vi "dropdown.vi"(9 "side":enum16{"l", "r"}(ring)) -> ()   [LabVIEW 2017]
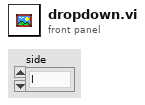
[diagram p1: front panel]
types:
  T1 = enum16{"hold", "f", "fl", "fr", "l", "r", "b", "bl", "br"}
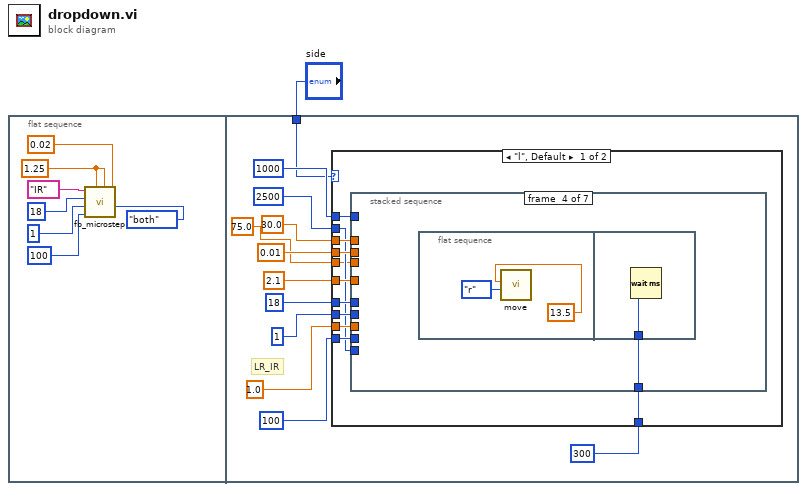
[diagram p0: block diagram]
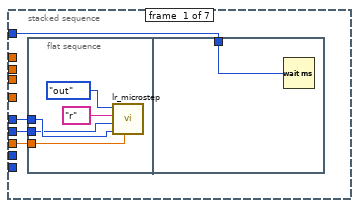
[diagram p2: hidden frame]
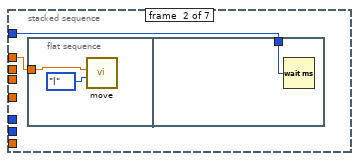
[diagram p3: hidden frame]
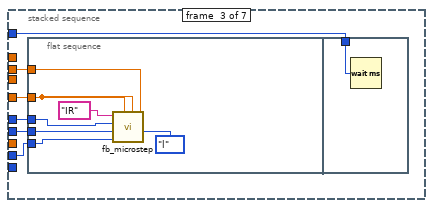
[diagram p4: hidden frame]
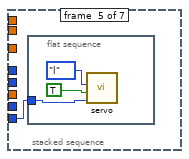
[diagram p5: hidden frame]
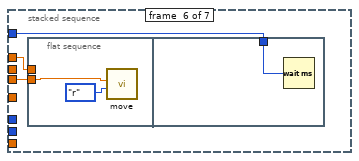
[diagram p6: hidden frame]
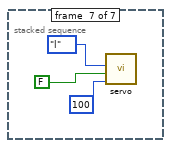
[diagram p7: hidden frame]
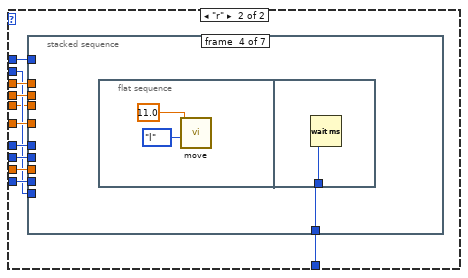
[diagram p8: hidden frame]
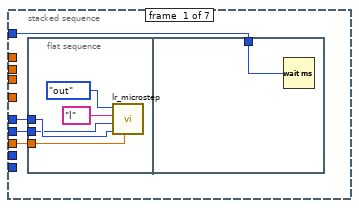
[diagram p9: hidden frame]
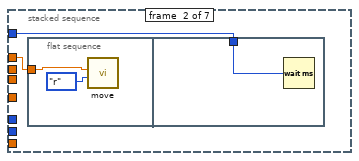
[diagram p10: hidden frame]
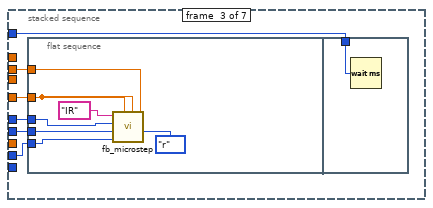
[diagram p11: hidden frame]
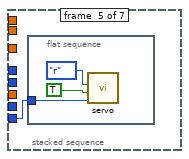
[diagram p12: hidden frame]
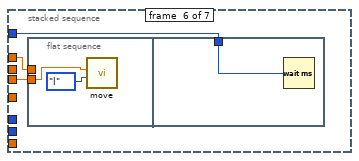
[diagram p13: hidden frame]
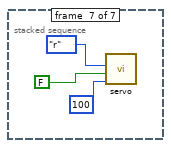
[diagram p14: hidden frame]
diagram:
  n1 = flat-sequence {
    tunnel: "side" -> [w11]
    frame #0 {
      w8 = 1.25 ("taget_IR_R")
      n2 = call "fb_microstep.vi"("Sensor"=enum16{"l", "r", "both"}."both", "precision"=0.02, "taget_IR_L"=w8, "taget_IR_R"=w8, "SamplingNUM"=100, "Step"=1, "Delay"=18, "Stop Mode"="IR") -> ()  [unwired: 3 in, 1 out]
    }
    frame #1 {
      # "LR_IR"
      n3 = case shown="\"l\", Default" w11 {
        tunnel: 18 ("Delay") -> [w31 w88]
        tunnel: 1 ("Step") -> [w30 w87]
        tunnel: 1.0 ("logic_num") -> [w29 w86]
        tunnel: 30.0 ("D") -> [w28 w85]
        tunnel: 2.1 ("taget_IR_R") -> [w27 w84]
        tunnel: 0.01 ("precision") -> [w26 w83]
        tunnel: 100 ("SamplingNUM") -> [w25 w82]
        tunnel: u32 1000 ("milliseconds to wait") -> [w24 w81]
        tunnel: u32 2500 ("delay") -> [w23 w80]
        tunnel: u32 300 ("milliseconds to wait") -> [w22 w79]
        tunnel: 75.0 ("D") -> [w21 w78]
        frame "l", Default {
          n4 = stacked-sequence {
            tunnel: w31 -> [w35 _ w50 _ _ _ _]
            tunnel: w30 -> [w34 _ w49 _ _ _ _]
            tunnel: w29 -> [w33 _ _ _ _ _ _]
            tunnel: w28 -> [_ w43 _ _ _ w71 _]
            tunnel: w27 -> [_ _ w52 _ _ _ _]
            tunnel: w26 -> [_ _ w51 _ _ _ _]
            tunnel: w25 -> [_ _ w48 _ _ _ _]
            tunnel: w24 -> [w32 w42 w47 _ _ w70 _]
            tunnel: w23 -> [_ _ _ _ w65 _ _]
            tunnel: w22 -> [_ _ _ w61 _ _ _]
            tunnel: w21 -> [_ _ _ _ _ w69 _]
            frame #0 {
              n5 = flat-sequence {
                tunnel: w35 -> [w38]
                tunnel: w34 -> [w37]
                tunnel: w33 -> [w36]
                tunnel: w32 -> [w41]
                frame #0 {
                  n6 = call "lr_microstep.vi"("target_IR"=w36, "Delay"=w38, "Step"=w37, "Stop Mode"="r", "IN-OUT"=enum16{"out", "in"}."out") -> ()  [unwired: 6 in, 1 out]
                }
                frame #1 {
                  n7 = Wait (ms)(milliseconds to wait=w41) -> ()  [unwired: 1 out]
                }
              }
            }
            frame #1 {
              n8 = flat-sequence {
                tunnel: w43 -> [w44]
                tunnel: w42 -> [w46]
                frame #0 {
                  n9 = call "move.vi"("Enum"=T1."l", "D"=w44) -> ()  [unwired: 10 in]
                }
                frame #1 {
                  n10 = Wait (ms)(milliseconds to wait=w46) -> ()  [unwired: 1 out]
                }
              }
            }
            frame #2 {
              n11 = flat-sequence {
                tunnel: w52 -> [w57]
                tunnel: w51 -> [w56]
                tunnel: w50 -> [w55]
                tunnel: w49 -> [w54]
                tunnel: w48 -> [w53]
                tunnel: w47 -> [w60]
                frame #0 {
                  n12 = call "fb_microstep.vi"("Sensor"=enum16{"l", "r", "both"}."l", "precision"=w56, "taget_IR_L"=w57, "taget_IR_R"=w57, "SamplingNUM"=w53, "Step"=w54, "Delay"=w55, "Stop Mode"="IR") -> ()  [unwired: 3 in, 1 out]
                }
                frame #1 {
                  n13 = Wait (ms)(milliseconds to wait=w60) -> ()  [unwired: 1 out]
                }
              }
            }
            frame #3 {
              n14 = flat-sequence {
                tunnel: w61 -> [w64]
                frame #0 {
                  n15 = call "move.vi"("Enum"=T1."r", "D"=13.5) -> ()  [unwired: 10 in]
                }
                frame #1 {
                  n16 = Wait (ms)(milliseconds to wait=w64) -> ()  [unwired: 1 out]
                }
              }
            }
            frame #4 {
              n17 = flat-sequence {
                tunnel: w65 -> [w66]
                frame #0 {
                  n18 = call "servo.vi"("delay"=w66, "in=true\nout = false"=TRUE ("in=true\nout = false"), "left-right"=enum16{"r", "l"}."l") -> ()  [unwired: 9 in]
                }
              }
            }
            frame #5 {
              n19 = flat-sequence {
                tunnel: w71 -> [_]
                tunnel: w69 -> [w72]
                tunnel: w70 -> [w74]
                frame #0 {
                  n20 = call "move.vi"("Enum"=T1."r", "D"=w72) -> ()  [unwired: 10 in]
                }
                frame #1 {
                  n21 = Wait (ms)(milliseconds to wait=w74) -> ()  [unwired: 1 out]
                }
              }
            }
            frame #6 {
              n22 = call "servo.vi"("delay"=u32 100, "in=true\nout = false"=FALSE ("in=true\nout = false"), "left-right"=enum16{"r", "l"}."l") -> ()  [unwired: 9 in]
            }
          }
        }
        frame "r" {
          n23 = stacked-sequence {
            tunnel: w88 -> [w92 _ w107 _ _ _ _]
            tunnel: w87 -> [w91 _ w106 _ _ _ _]
            tunnel: w86 -> [w90 _ _ _ _ _ _]
            tunnel: w85 -> [_ w100 _ _ _ w128 _]
            tunnel: w84 -> [_ _ w109 _ _ _ _]
            tunnel: w83 -> [_ _ w108 _ _ _ _]
            tunnel: w82 -> [_ _ w105 _ _ _ _]
            tunnel: w81 -> [w89 w99 w104 _ _ w127 _]
            tunnel: w80 -> [_ _ _ _ w122 _ _]
            tunnel: w79 -> [_ _ _ w118 _ _ _]
            tunnel: w78 -> [_ _ _ _ _ w126 _]
            frame #0 {
              n24 = flat-sequence {
                tunnel: w92 -> [w95]
                tunnel: w91 -> [w94]
                tunnel: w90 -> [w93]
                tunnel: w89 -> [w98]
                frame #0 {
                  n25 = call "lr_microstep.vi"("target_IR"=w93, "Delay"=w95, "Step"=w94, "Stop Mode"="l", "IN-OUT"=enum16{"out", "in"}."out") -> ()  [unwired: 6 in, 1 out]
                }
                frame #1 {
                  n26 = Wait (ms)(milliseconds to wait=w98) -> ()  [unwired: 1 out]
                }
              }
            }
            frame #1 {
              n27 = flat-sequence {
                tunnel: w100 -> [w102]
                tunnel: w99 -> [w103]
                frame #0 {
                  n28 = call "move.vi"("Enum"=T1."r", "D"=w102) -> ()  [unwired: 10 in]
                }
                frame #1 {
                  n29 = Wait (ms)(milliseconds to wait=w103) -> ()  [unwired: 1 out]
                }
              }
            }
            frame #2 {
              n30 = flat-sequence {
                tunnel: w109 -> [w114]
                tunnel: w108 -> [w113]
                tunnel: w107 -> [w112]
                tunnel: w106 -> [w111]
                tunnel: w105 -> [w110]
                tunnel: w104 -> [w117]
                frame #0 {
                  n31 = call "fb_microstep.vi"("Sensor"=enum16{"l", "r", "both"}."r", "precision"=w113, "taget_IR_L"=w114, "taget_IR_R"=w114, "SamplingNUM"=w110, "Step"=w111, "Delay"=w112, "Stop Mode"="IR") -> ()  [unwired: 3 in, 1 out]
                }
                frame #1 {
                  n32 = Wait (ms)(milliseconds to wait=w117) -> ()  [unwired: 1 out]
                }
              }
            }
            frame #3 {
              n33 = flat-sequence {
                tunnel: w118 -> [w121]
                frame #0 {
                  n34 = call "move.vi"("Enum"=T1."l", "D"=11.0) -> ()  [unwired: 10 in]
                }
                frame #1 {
                  n35 = Wait (ms)(milliseconds to wait=w121) -> ()  [unwired: 1 out]
                }
              }
            }
            frame #4 {
              n36 = flat-sequence {
                tunnel: w122 -> [w123]
                frame #0 {
                  n37 = call "servo.vi"("delay"=w123, "in=true\nout = false"=TRUE ("in=true\nout = false"), "left-right"=enum16{"r", "l"}."r") -> ()  [unwired: 9 in]
                }
              }
            }
            frame #5 {
              n38 = flat-sequence {
                tunnel: w128 -> [_]
                tunnel: w126 -> [w129]
                tunnel: w127 -> [w131]
                frame #0 {
                  n39 = call "move.vi"("Enum"=T1."l", "D"=w129) -> ()  [unwired: 10 in]
                }
                frame #1 {
                  n40 = Wait (ms)(milliseconds to wait=w131) -> ()  [unwired: 1 out]
                }
              }
            }
            frame #6 {
              n41 = call "servo.vi"("delay"=u32 100, "in=true\nout = false"=FALSE ("in=true\nout = false"), "left-right"=enum16{"r", "l"}."r") -> ()  [unwired: 9 in]
            }
          }
        }
      }
    }
  }
